vi "Caterpillar Tester.vi"() -> ()   [LabVIEW 2012]
uses:
  <vilib>/Rock Robotics/WPI/Solenoid/WPI_SolenoidValue.ctl
panel:
  out "Back Leg Cmd":bool
  out "Mid Leg Cmd":enum16{"Down Closed", "Down Opened", "Up"}(ring)=enum."Down Opened"
  out "Mid Foot":T1=enum."Forward"
  in  "Back Leg PS":bool=TRUE
  out "Skids":bool
  out "Front Leg Cmd":enum16{"Down Closed", "Down Opened", "Up"}(ring)=enum."Down Opened"
  in  "Mid Claw Cmd":bool
  in  "Front Leg Up":bool
  out "Old state 2":string
  out "old state 0":string
  out "Old state 1":string
  in  "Front Claw Cmd":bool
  out "Mid Claw":T1=enum."Forward"
  out "Back Claw":T1=enum."Forward"
  out "Front Foot":T1=enum."Forward"
  out "Front Claw":T1=enum."Forward"
  out "Current  State":string
  in  "Back Leg Up":bool
  in  "Mid Leg Up":bool
  in  "Mid Leg PS":bool=TRUE
  in  "Front Leg PS":bool=TRUE
  # "Using the Caterpillar Tester\n\nSetup:\n1) Make sure deploy target is set to\n     Main Application Instance or My Computer\n2) Go to Edit menu and click on \n     Reinitialize Values to Default\n2) Click the Run Continuously button\n\nError-Free Climbing:\n1) Click on A (Front Claw Cmd)\n2) Click on B (Mid Claw Cmd)\n3) Turn off Front Leg PS button\n4) Turn on Front Leg Up button\n5) Turn on Front Leg PS button\n6) Turn off Front Leg Up button\n7) Turn off Mid Leg PS button\n8) Turn on Mid Leg Up button\n9) Turn on Mid Leg PS button\n10) Turn off Mid Leg Up button\n11) Turn off Back Leg PS button\n12) Turn on Back Leg Up button\n13) Turn on Back Leg PS button\n14) Turn off Back Leg Up button\n\nAll legs are now across first horizontal pole.\nRepeat steps 3 through 14 to cross the\nsecond horizontal pole for a 30-point climb!"
  # "Proximity sensors (On == Not sensing corner)"
  # "Limit\nswitches\nfor\nlegs\n(On \n==\nLeg\nis\nUP)"
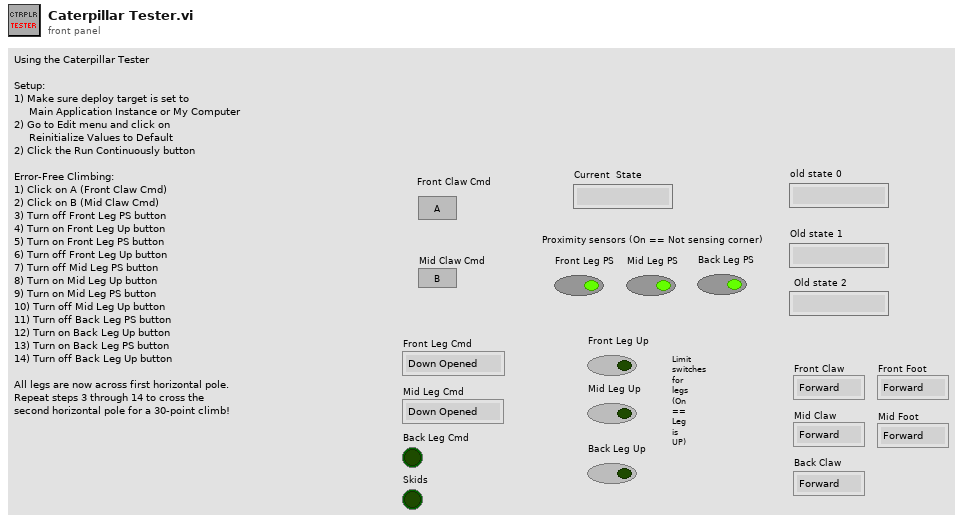
[diagram p1: front panel]
types:
  T1 = typedef "WPI_SolenoidValue.ctl" = enum16{"Off", "On", "Forward", "Reverse"}
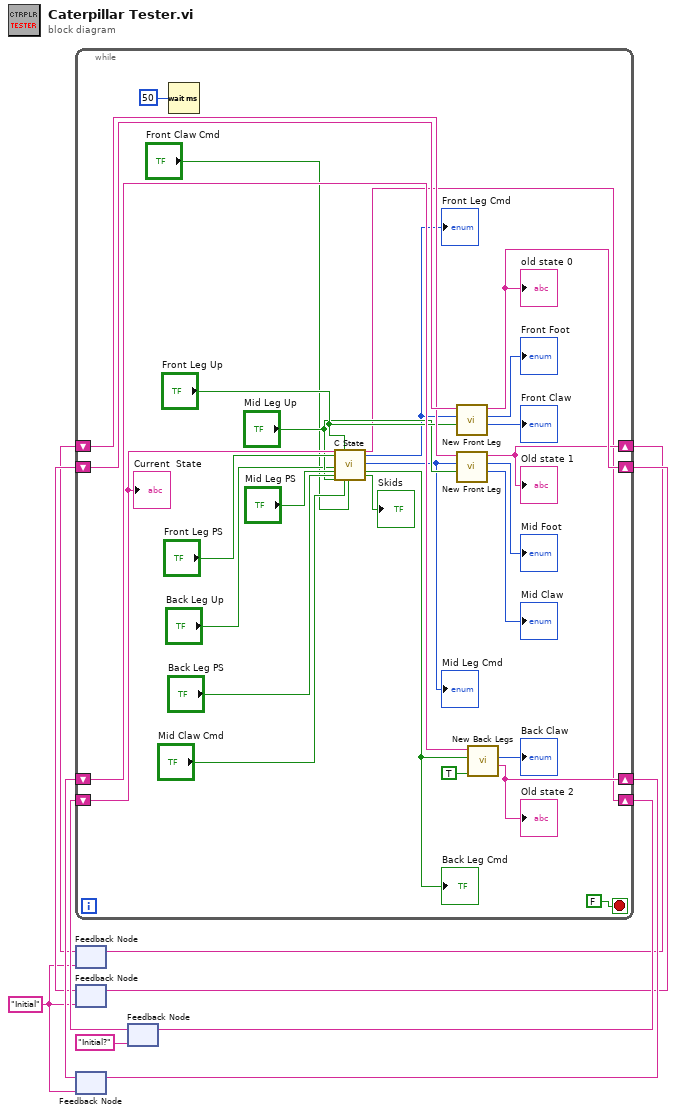
[diagram p0: block diagram]
diagram:
  w1 = "Initial" ("Old state")
  n1 = feedback #1(w1) -> (w2:string)
  n2 = feedback #2(w1) -> (w4:string)
  n3 = feedback #3(w1) -> (w6:string)
  n4 = feedback #4("Initial?" ("New State")) -> (w9:string)
  n5 = while {
    shift-right: [w13] -> w10
    shift-left: w9 -> [w21]
    shift-right: [w30] -> w7
    shift-left: w6 -> [w33]
    shift-right: [w31] -> w5
    shift-left: w4 -> [w32]
    shift-right: [w27] -> w3
    shift-left: w2 -> [w28]
    stop <- FALSE stop-if-true
    n6 = Wait (ms)(milliseconds to wait=u32 50) -> ()  [unwired: 1 out]
    n7 = call "C State.vi"("State"=w21, "Front Leg PS"="Front Leg PS", "Back Leg Up"="Back Leg Up", "Mid Leg PS"="Mid Leg PS", "Back Leg PS"="Back Leg PS", "Mid Leg Up"="Mid Leg Up", "Front Leg Up"="Front Leg Up", "Back Claws Cmd"="Mid Claw Cmd", "Front Claw Cmd"="Front Claw Cmd") -> ("newState"=w13:string, "Front Leg Cmd"=w11:enum16{"Down Closed", "Down Opened", "Up"}, "Mid Leg Cmd"=w12:enum16{"Down Closed", "Down Opened", "Up"}, "Engage Back Leg"=w15:bool, "Skids"=→"Skids":bool)  [unwired: 13 in, 1 out]
    "Front Leg Cmd" <- w11
    "Mid Leg Cmd" <- w12
    "Back Leg Cmd" <- w15
    n8 = call "New Front Leg.vi"("Leg up"="Front Leg Up", "Command"=w11, "Old State"=w32) -> ("Claw"=→"Front Claw":T1, "Foot"=→"Front Foot":T1, "New state"=w31:string)  [unwired: 6 in]
    "old state 0" <- w31
    n9 = call "New Front Leg.vi"("Leg up"="Mid Leg Up", "Command"=w12, "Old State"=w28) -> ("Claw"=→"Mid Claw":T1, "Foot"=→"Mid Foot":T1, "New state"=w27:string)  [unwired: 6 in]
    "Old state 1" <- w27
    n10 = call "New Back Legs.vi"("isDualActing"=TRUE, "Engage Leg 1/2"=w15, "New state"=w33) -> ("Old state"=w30:string, "Claw"=→"Back Claw":T1)  [unwired: 7 in]
    "Old state 2" <- w30
    "Current  State" <- w21
  }
  n11 = feedback-in #1(w3) -> ()
  n12 = feedback-in #2(w5) -> ()
  n13 = feedback-in #3(w7) -> ()
  n14 = feedback-in #4(w10) -> ()
